vi "total_valve_control.vi"() -> ()   [LabVIEW 2014]
panel:
  in  "Read pressures?":bool
  out "Valve 2 Closed?":bool
  out "Valve 1 Closed?":bool
  out "Valve 3 Closed?":bool
  out "Cold Cathode Gauge Pressure [Torr]":dbl format="%_3g"
  out "Valve Percentage Open":dbl
  out "Unacceptable Flow Rate Value":bool
  in  "Enter Flow Rate (mbar*Liters/sec)":dbl
  out "Pirani Gauge Pressure [Torr]":dbl format="%_3g"
  out "Valve 2 Open?":bool
  out "Valve 2, value 2":dbl format="%0.2f"
  out "Valve 2, value 1":dbl format="%0.2f"
  out "Valve 1, value 2":dbl format="%0.2f"
  out "Valve 1, value 1":dbl format="%0.2f"
  out "Valve 3, value 2":dbl format="%0.2f"
  out "Valve 3, value 1":dbl format="%0.2f"
  in  "?":bool
  out "Valve 3 Open?":bool
  out "Valve 1 Open?":bool
  in  "Open Valve 2?":bool
  in  "Open Valve 3?":bool
  in  "Open Valve 1?":bool
  # "ROUGHING\nPUMP"
  # "Valve 1"
  # "Valve 3"
  # "TURBO"
  # "Valve 2"
  # "Vent Valve"
  # "CHAMBER"
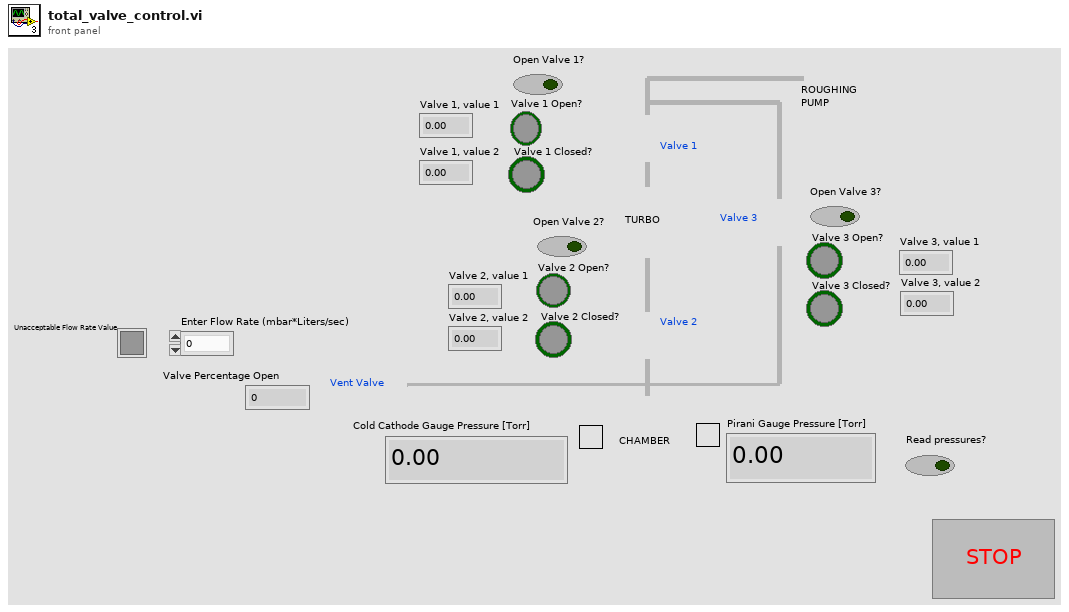
[diagram p1: front panel]
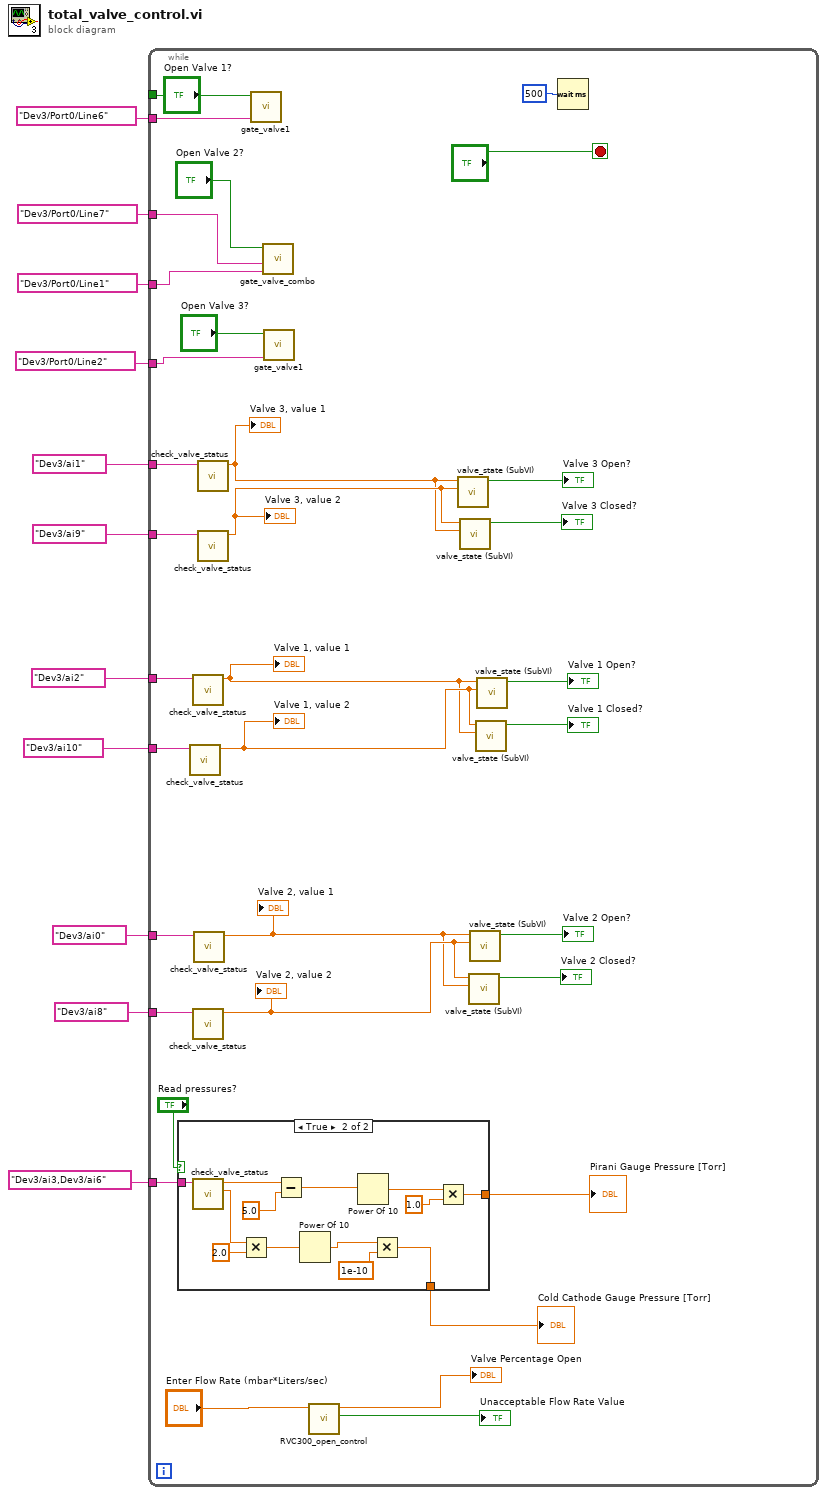
[diagram p0: block diagram]
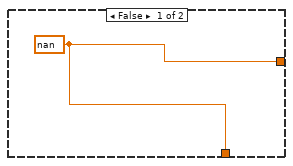
[diagram p2: hidden frame]
diagram:
  n1 = while {
    tunnel: tag "Dev3/ai2" ("Valve 1 Ch. 1") -> [w45]
    tunnel: tag "Dev3/ai10" ("Valve 1 Ch. 2") -> [w44]
    tunnel: tag "Dev3/ai1" ("Valve 3 Ch. 1") -> [w43]
    tunnel: tag "Dev3/ai9" ("Valve 3 Ch. 2") -> [w42]
    tunnel: ["Open Valve 1?"] -> _
    tunnel: tag "Dev3/Port0/Line6" ("Control Valve 1") -> [w40]
    tunnel: tag "Dev3/Port0/Line2" ("Control Valve  3") -> [w37]
    tunnel: tag "Dev3/Port0/Line7" ("Control Valve 2") -> [w38]
    tunnel: tag "Dev3/Port0/Line1" ("Channel for Valve Pair 2") -> [w39]
    tunnel: tag "Dev3/ai0" ("Channel 1") -> [w31]
    tunnel: tag "Dev3/ai8" ("Channel 1") -> [w30]
    tunnel: tag "Dev3/ai3,Dev3/ai6" ("Channel 1") -> [w29]
    stop <- "?" stop-if-true
    n2 = case shown="True" "Read pressures?" {
      tunnel: w29 -> [_ w59]
      tunnel: [w46 w53] -> w28
      tunnel: [w46 w47] -> w12
      frame False {
        w46 = nan
      }
      frame True {
        n3 = call "check_valve_status.vi"("Channel 1"=w59) -> ("Ch. 2 value"=w52:dbl, "Ch. 1 value"=w57:dbl)  [unwired: 9 in]
        n4 = Multiply(x=w52, y=2.0) -> (x*y=w50:dbl)
        n5 = Subtract(x=w57, y=5.0) -> (x-y=w56:dbl)
        n6 = Power Of 10(x=w50) -> (10^x=w49:dbl)
        n7 = Power Of 10(x=w56) -> (10^x=w55:dbl)
        n8 = Multiply(x=w49, y=1e-10) -> (x*y=w47:dbl)
        n9 = Multiply(x=w55, y=1.0) -> (x*y=w53:dbl)
      }
    }
    "Pirani Gauge Pressure [Torr]" <- w28
    "Cold Cathode Gauge Pressure [Torr]" <- w12
    n10 = call "check_valve_status.vi"("Channel 1"=w44) -> ("Ch. 1 value"=w20:dbl)  [unwired: 9 in, 1 out]
    "Valve 1, value 2" <- w20
    n11 = call "check_valve_status.vi"("Channel 1"=w45) -> ("Ch. 1 value"=w19:dbl)  [unwired: 9 in, 1 out]
    "Valve 1, value 1" <- w19
    n12 = call "check_valve_status.vi"("Channel 1"=w30) -> ("Ch. 1 value"=w17:dbl)  [unwired: 9 in, 1 out]
    "Valve 2, value 2" <- w17
    n13 = call "check_valve_status.vi"("Channel 1"=w31) -> ("Ch. 1 value"=w16:dbl)  [unwired: 9 in, 1 out]
    "Valve 2, value 1" <- w16
    n14 = call "check_valve_status.vi"("Channel 1"=w43) -> ("Ch. 1 value"=w23:dbl)  [unwired: 9 in, 1 out]
    "Valve 3, value 1" <- w23
    n15 = call "check_valve_status.vi"("Channel 1"=w42) -> ("Ch. 1 value"=w24:dbl)  [unwired: 9 in, 1 out]
    "Valve 3, value 2" <- w24
    n16 = call "gate_valve1.vi"("Open Valve?"="Open Valve 1?", "physical channels"=w40) -> ()  [unwired: 9 in]
    n17 = call "gate_valve_combo.vi"("Channel for Valve Pair 2"=w39, "Channel for Valve Pair 1"=w38, "Open Gate Valve?"="Open Valve 2?") -> ()  [unwired: 9 in]
    n18 = call "gate_valve1.vi"("Open Valve?"="Open Valve 3?", "physical channels"=w37) -> ()  [unwired: 9 in]
    n19 = call "RVC300_open_control.vi"("Enter Flow Rate (mbar*Liters/sec)"="Enter Flow Rate (mbar*Liters/sec)") -> ("Unacceptable Flow Rate Value"=→"Unacceptable Flow Rate Value":bool, "Valve Percentage Open"=→"Valve Percentage Open":dbl)  [unwired: 9 in]
    n20 = call "valve_state (SubVI).vi"("Ch. 1 value 2"=w24, "Ch. 1 value"=w23) -> ("Boolean"=→"Valve 3 Open?":bool)  [unwired: 9 in]
    n21 = call "valve_state (SubVI).vi"("Ch. 1 value 2"=w23, "Ch. 1 value"=w24) -> ("Boolean"=→"Valve 3 Closed?":bool)  [unwired: 9 in]
    n22 = call "valve_state (SubVI).vi"("Ch. 1 value 2"=w16, "Ch. 1 value"=w17) -> ("Boolean"=→"Valve 2 Closed?":bool)  [unwired: 9 in]
    n23 = call "valve_state (SubVI).vi"("Ch. 1 value 2"=w17, "Ch. 1 value"=w16) -> ("Boolean"=→"Valve 2 Open?":bool)  [unwired: 9 in]
    n24 = call "valve_state (SubVI).vi"("Ch. 1 value 2"=w19, "Ch. 1 value"=w20) -> ("Boolean"=→"Valve 1 Closed?":bool)  [unwired: 9 in]
    n25 = call "valve_state (SubVI).vi"("Ch. 1 value 2"=w20, "Ch. 1 value"=w19) -> ("Boolean"=→"Valve 1 Open?":bool)  [unwired: 9 in]
    n26 = Wait (ms)(milliseconds to wait=u32 500) -> ()  [unwired: 1 out]
  }
